vi "SetExtGain.vi"(3 "Gain":enum16{"1x", "8x", "64x"}(ring)=enum."64x", 4 "Device":u8=1, 5 "Serial port":refnum<visa-resource-name>) -> (1 "Device out":u8=1, 2 "Serial port out":refnum<visa-resource-name>)   [LabVIEW 2021]
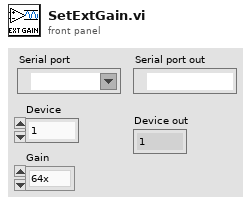
[diagram p1: front panel]
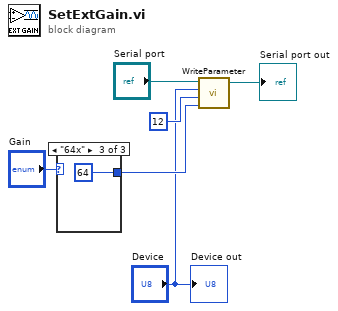
[diagram p0: block diagram]
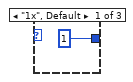
[diagram p2: hidden frame]
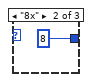
[diagram p3: hidden frame]
diagram:
  n1 = case shown="\"64x\"" "Gain" {
    tunnel: [1 8 64] -> w2
    frame "1x", Default {
    }
    frame "8x" {
    }
    frame "64x" {
    }
  }
  n2 = call "WriteParameter.vi"("Value"=w2, "Address"=u32 12, "Device"="Device", "Serial port"="Serial port") -> ("Serial port out"=→"Serial port out":refnum<visa-resource-name>)  [unwired: 2 in]
  "Device out" <- "Device"
